vi "RegExTest.vi"() -> ()   [LabVIEW 2016, in "M1M3SupportEUI_Views.lvlib"]
uses:
  M1M3SupportEUI_Views.lvlib
panel:
  in  "\"reg ex\"":string
  out "EndString":string
  out "MiddleString":string
  out "BeginningString":string
  in  "The String":string
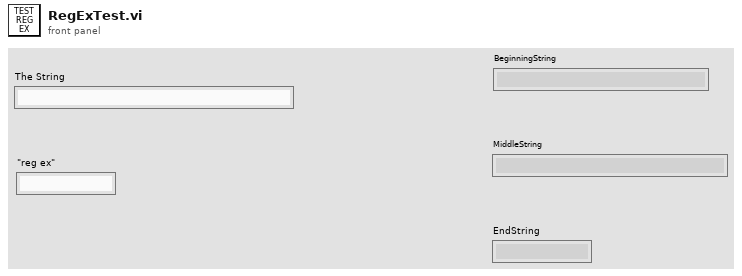
[diagram p1: front panel]
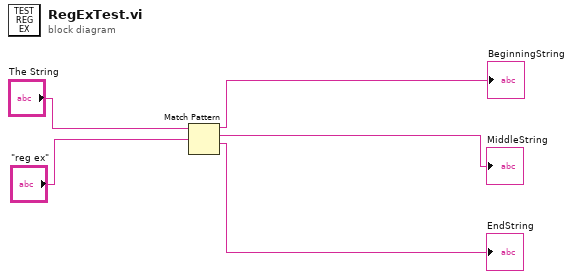
[diagram p0: block diagram]
diagram:
  n1 = Match Pattern(string="The String", regular expression="\"reg ex\"") -> (before substring=→"BeginningString":string, match substring=→"MiddleString":string, after substring=→"EndString":string)  [unwired: 1 in, 1 out]
